vi "Get Time.vi"() -> (3 "time":string)   [LabVIEW 2025, in "Full User Interface.lvlib"]
uses:
  Full User Interface.lvlib
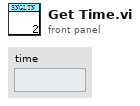
[diagram p1: front panel]
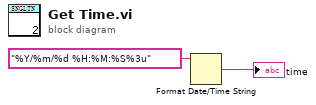
[diagram p0: block diagram]
diagram:
  n1 = Format Date/Time String(time format string (%c)="%Y/%m/%d %H:%M:%S%3u") -> (date/time string=→"time":string)  [unwired: 2 in]
